vi "Give.vi"(8 "error in (no error)":errorcluster caption="entrée d'erreur (pas d'erreur)", 11 "A en entrée":refnum<class "A.lvclass">) -> (0 "error out":errorcluster caption="sortie d'erreur", 3 "A en sortie":refnum<class "A.lvclass">)   [LabVIEW 2015, in "A.lvclass"]
uses:
  A.lvclass
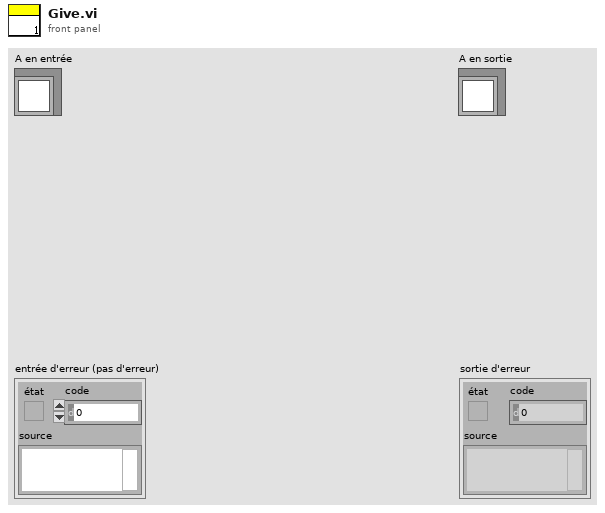
[diagram p1: front panel]
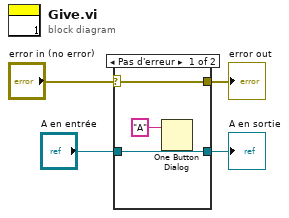
[diagram p0: block diagram]
diagram:
  n1 = case shown="Pas d'erreur" "error in (no error)" {
    selector: "error in (no error)" -> [w6 w9]
    tunnel: [w7 w8] -> w3
    tunnel: "A en entrée" -> [w7 w8]
    tunnel: [w6 w9] -> w1
    frame No Error {
      n2 = One Button Dialog(message="A") -> ()  [unwired: 1 in, 1 out]
    }
    frame Error {
    }
  }
  "error out" <- w1
  "A en sortie" <- w3
